vi "Update Wavenet-IIR.vi"(1 "Wavenet-IIR Gradients":T3 {"Forwards, D" format="%.3f"; "Feedbacks, C" format="%.3f"; "Weights, W" format="%.3f"; "Shifts, B" format="%.3f"; "Scales, A" format="%.3f"}, 2 "Wavenet-IIR Older":T2 {"Function, dy" format="%.3f"; "Function, y" format="%.3f"; "Tau, t" format="%.3f"; "Forwards, D" format="%.3f"; "Feedbacks, C" format="%.3f"; "Weights, W" format="%.3f"; "Shifts, B" format="%.3f"; "Scales, A" format="%.3f"}, 3 "Wavenet-IIR Parameters":T1={"Activation function, fn"=0, "Neurons, J"=1, "Feedbacks, Q"=1, "Feedforwards, R"=1, "Inputs, I"=1, "Outputs, P"=1, "Weights, hW"=0.0, "Feedbacks, ha"=0.0, "Forwards, hb"=0.0, "Scalings, hA"=0.0, "Shiftings, hB"=0.0, "Persistant signal, ps"=0.0} {"Persistant signal, ps" format="%.2e"; "Shiftings, hB" format="%.2e"; "Scalings, hA" format="%.2e"; "Forwards, hb" format="%.2e"; "Feedbacks, ha" format="%.2e"; "Weights, hW" format="%.2e"; "Outputs, P" min=1 max=10 step=1; "Inputs, I" min=1 max=10 step=1; "Feedforwards, R" min=1 max=10 step=1; "Feedbacks, Q" min=1 max=10 step=1; "Neurons, J" min=1 max=10 step=1; "Activation function, fn" items=["Morlet", "RASP1", "RASP2", "RASP3", "POLYWOG1", "POLYWOG2", "POLYWOG3", "POLYWOG4", "POLYWOG5", "Shannon", "Atomic", "Flat top 1", "Flat top 2", "Flat top 3", "Flat top 4", "Flat top 5", "Flat top 6", "Hanning", "Hamming", "Blackman", "Blackman-Harris"]}) -> (0 "Wavenet-IIR New":T2 {"Function, dy" format="%.3f"; "Function, y" format="%.3f"; "Tau, t" format="%.3f"; "Forwards, D" format="%.3f"; "Feedbacks, C" format="%.3f"; "Weights, W" format="%.3f"; "Shifts, B" format="%.3f"; "Scales, A" format="%.3f"})   [LabVIEW 2022 SP3]
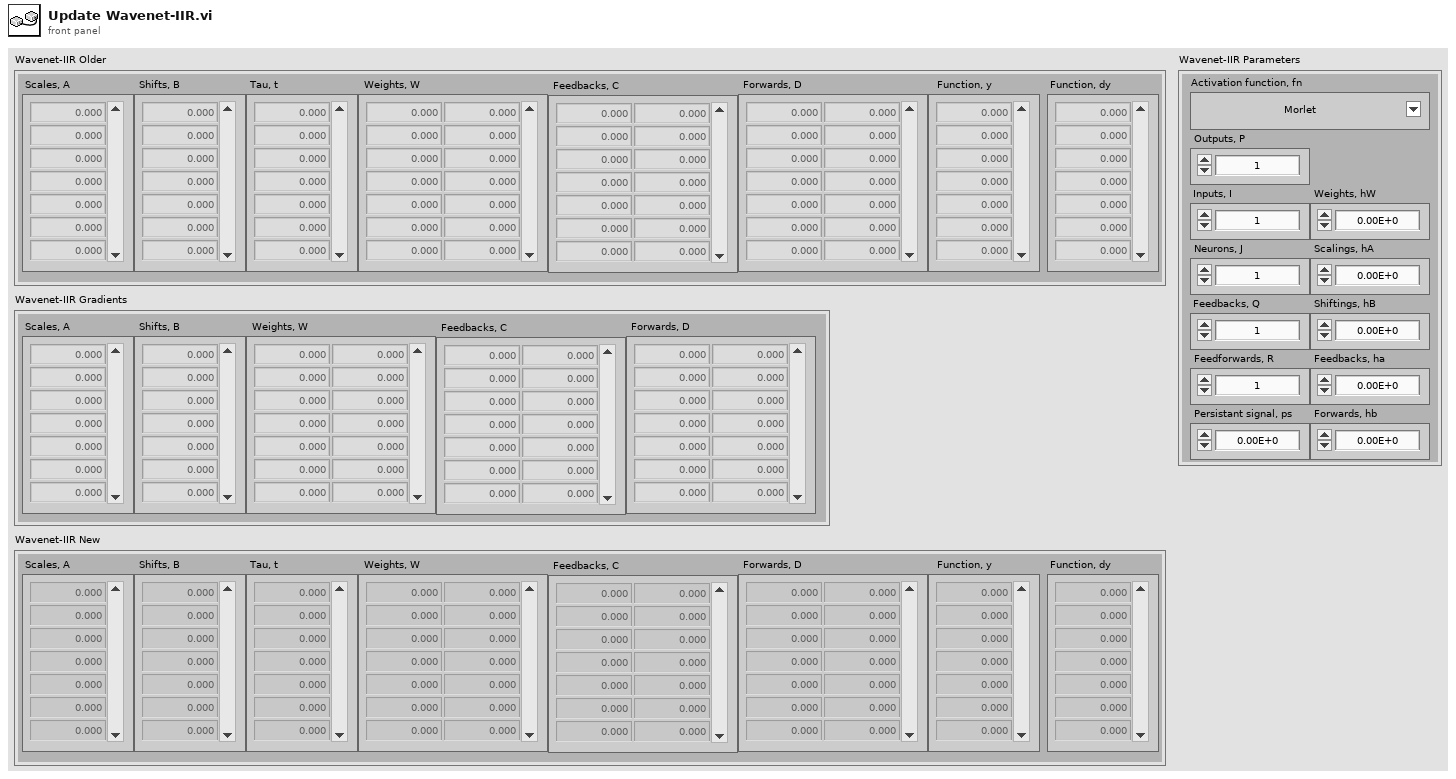
[diagram p1: front panel]
types:
  T1 = cluster{"Activation function, fn":u16, "Neurons, J":i32, "Feedbacks, Q":i32, "Feedforwards, R":i32, "Inputs, I":i32, "Outputs, P":i32, "Weights, hW":dbl, "Feedbacks, ha":dbl, "Forwards, hb":dbl, "Scalings, hA":dbl, "Shiftings, hB":dbl, "Persistant signal, ps":dbl}
  T2 = cluster{"Scales, A":dbl[], "Shifts, B":dbl[], "Weights, W":dbl[][], "Feedbacks, C":dbl[][], "Forwards, D":dbl[][], "Tau, t":dbl[], "Function, y":dbl[], "Function, dy":dbl[]}
  T3 = cluster{"Scales, A":dbl[], "Shifts, B":dbl[], "Weights, W":dbl[][], "Feedbacks, C":dbl[][], "Forwards, D":dbl[][]}
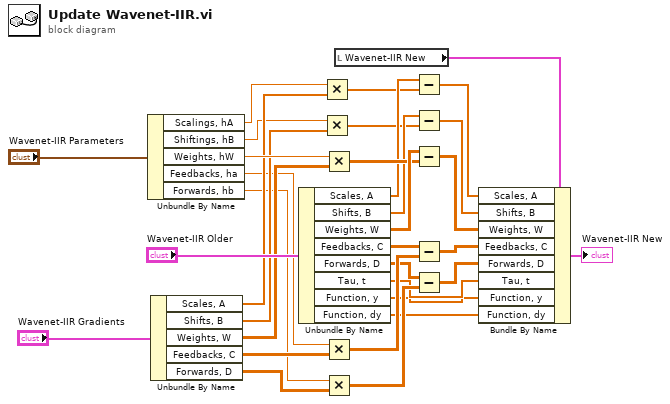
[diagram p0: block diagram]
diagram:
  n1 = Unbundle By Name("Wavenet-IIR Parameters") -> ("Scalings, hA"=w22:dbl, "Shiftings, hB"=w14:dbl, "Weights, hW"=w25:dbl, "Feedbacks, ha"=w9:dbl, "Forwards, hb"=w5:dbl)
  n2 = Unbundle By Name("Wavenet-IIR Gradients") -> ("Scales, A"=w21:dbl[], "Shifts, B"=w15:dbl[], "Weights, W"=w29:dbl[][], "Feedbacks, C"=w10:dbl[][], "Forwards, D"=w4:dbl[][])
  n3 = Unbundle By Name("Wavenet-IIR Older") -> ("Scales, A"=w24:dbl[], "Shifts, B"=w17:dbl[], "Weights, W"=w30:dbl[][], "Feedbacks, C"=w12:dbl[][], "Forwards, D"=w6:dbl[][], "Tau, t"=w3:dbl[], "Function, y"=w2:dbl[], "Function, dy"=w1:dbl[])
  n4 = Multiply(x=w22, y=w21) -> (x*y=w23:dbl[])
  n5 = Multiply(x=w14, y=w15) -> (x*y=w16:dbl[])
  n6 = Multiply(x=w25, y=w29) -> (x*y=w28:dbl[][])
  n7 = Multiply(x=w9, y=w10) -> (x*y=w11:dbl[][])
  n8 = Multiply(x=w5, y=w4) -> (x*y=w7:dbl[][])
  n9 = local read "Wavenet-IIR New"() -> (w27:T2)
  n10 = Subtract(x=w24, y=w23) -> (x-y=w20:dbl[])
  n11 = Subtract(x=w17, y=w16) -> (x-y=w18:dbl[])
  n12 = Subtract(x=w30, y=w28) -> (x-y=w19:dbl[][])
  n13 = Subtract(x=w12, y=w11) -> (x-y=w13:dbl[][])
  n14 = Subtract(x=w6, y=w7) -> (x-y=w8:dbl[][])
  n15 = Bundle By Name(cluster=w27, "Scales, A"=w20, "Shifts, B"=w18, "Weights, W"=w19, "Feedbacks, C"=w13, "Forwards, D"=w8, "Tau, t"=w3, "Function, y"=w2, "Function, dy"=w1) -> (→"Wavenet-IIR New":T2)
